vi "HeartRateControl_SMC+FF_New_Int.vi"() -> ()   [LabVIEW 2013]
uses:
  <vilib>/Instr/_visa.llb/VISA Configure Serial Port (Instr).vi
panel:
  out "Volt2":dbl
  out "Volt":dbl
  out "TM":dbl
  out "Torque [Nm]":dbl
  out "Cadence [rpm]":dbl
  out "Power [W]":dbl
  in  "file path":path
  out "Heart Rate [bpm]":u32
  out "Heart Rate [bpm]":dbl(knob) scale=0.0..220.0
  in  "VISA resource name":refnum<visa-resource-name>="COM1"
  out "Power [W]":dbl(slide) scale=0.0..250.0
  out "Cadence [rpm]":dbl(knob) scale=0.0..120.0
  out "Count":dbl
  out "Torque [Nm]":dbl(knob) scale=-250.0..250.0
  out "Torque [V]":dbl
  out "Sine":bool
  out "Cosine":bool
  in  "stop (F)":bool caption="Stop"
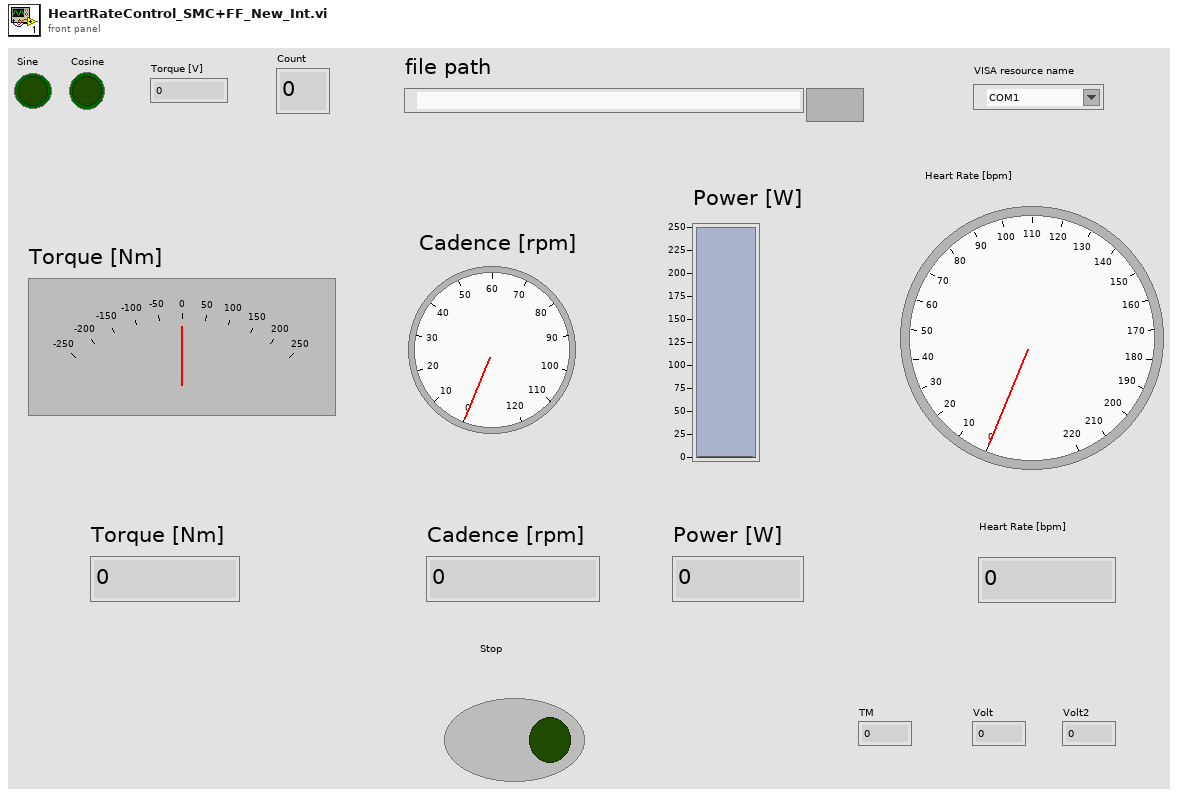
[diagram p1: front panel]
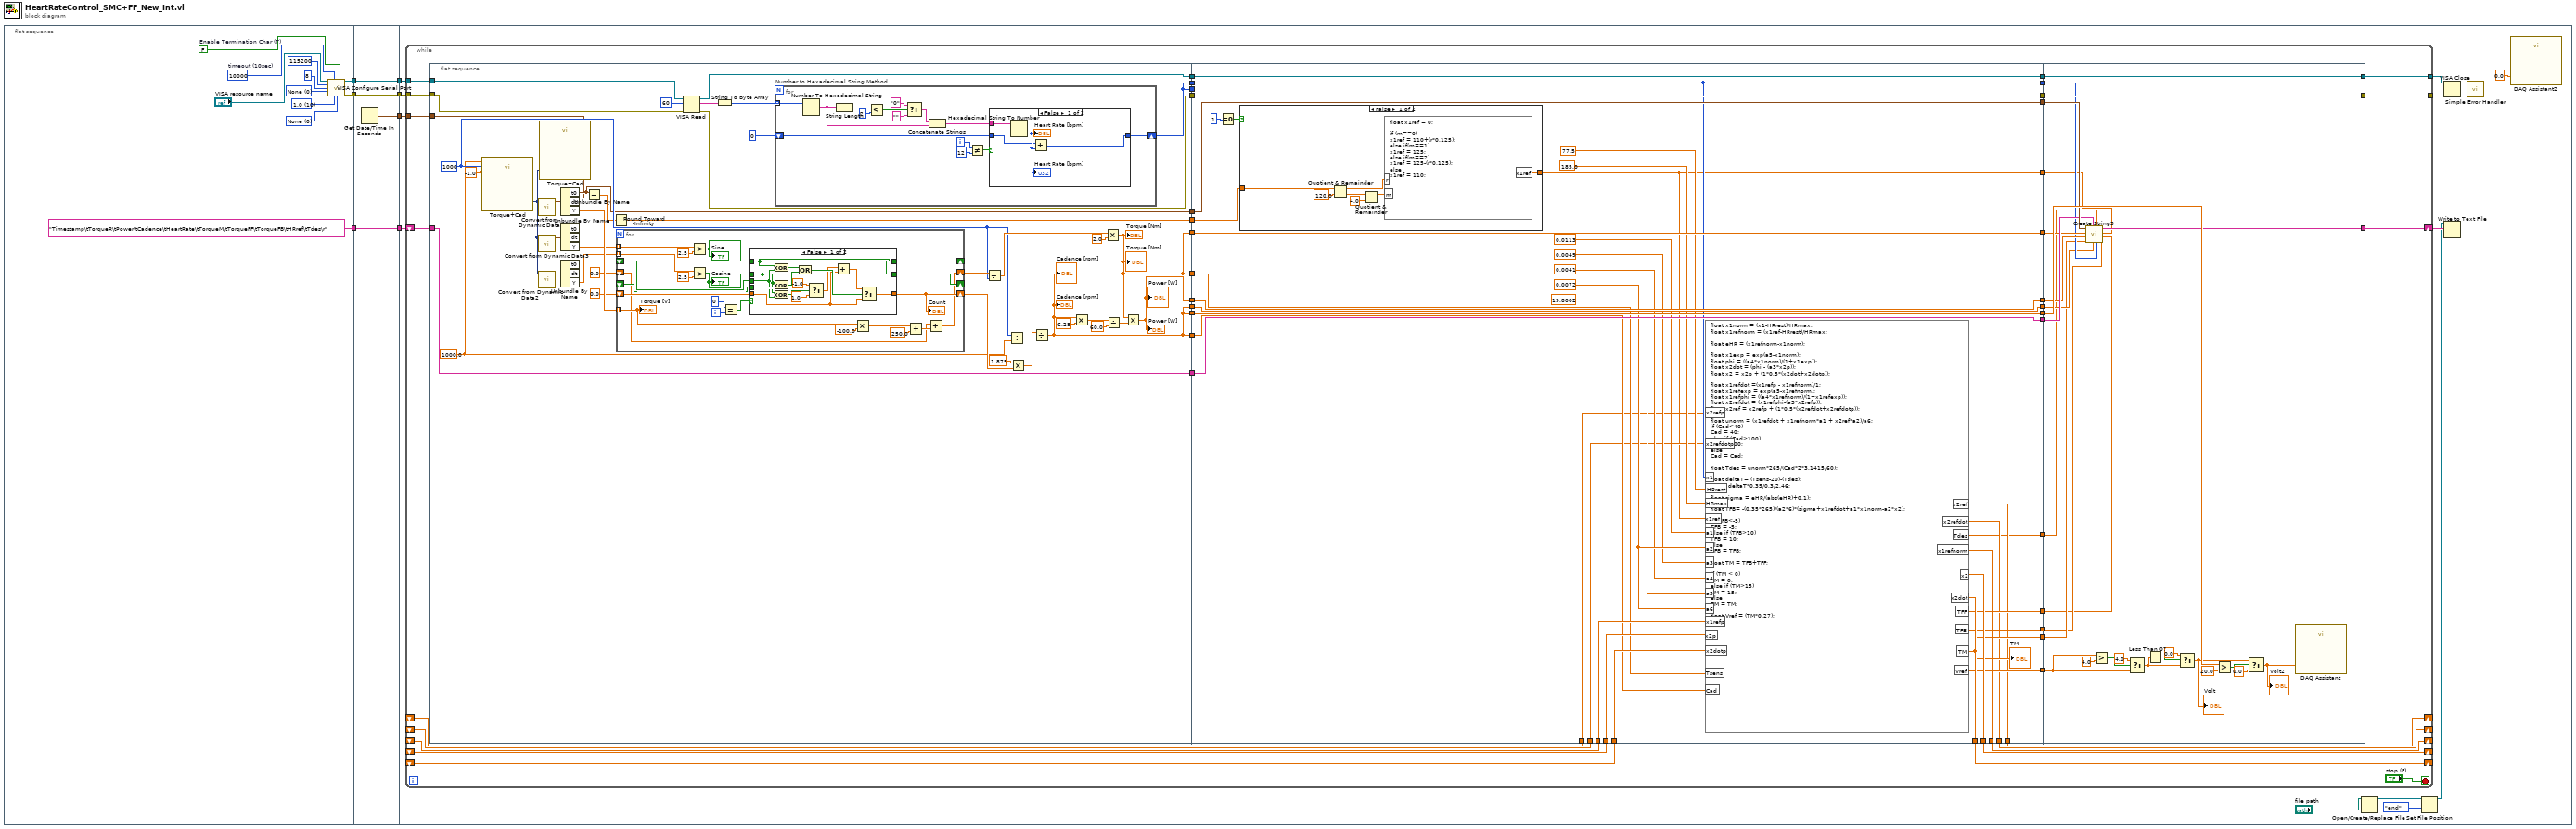
[diagram p0: block diagram]
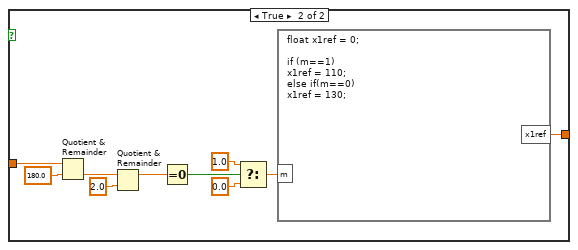
[diagram p4: hidden frame]
diagram:
  n1 = flat-sequence {
    tunnel: [w10] -> w6
    tunnel: [w9] -> w4
    tunnel: ["Timestamp\tTorqueR\tPower\tCadence\tHeartRate\tTorqueM\tTorqueFF\tTorqueFB\tHRref\tTdes\r" ("String out")] -> w2
    tunnel: [w22] -> w7
    tunnel: w6 -> [w22]
    tunnel: [w21] -> w5
    tunnel: w4 -> [w21]
    tunnel: [w20] -> w3
    tunnel: w2 -> [w20]
    tunnel: [w19] -> w1
    tunnel: w7 -> [w26]
    tunnel: w5 -> [w25]
    tunnel: w3 -> [w24]
    tunnel: w1 -> [w23]
    frame #0 {
      w16 = u16 0 items=["None"=0, "XON/XOFF"=1, "RTS/CTS"=2, "DTR/DSR"=4] ("flow control")
      w15 = u16 10 items=["1.0"=10, "1.5"=15, "2.0"=20] ("stop bits")
      w12 = u16 0 items=["None", "Odd", "Even", "Mark", "Space"] ("parity")
      w14 = FALSE  # Enable Termination Char (T)
      w13 = u32 10000  # timeout (10sec)
      n2 = call-poly "VISA Configure Serial Port"("VISA resource name"="VISA resource name", "timeout (10sec)"=w13, "Enable Termination\nChar (T)"=w14, "baud rate (9600)"=u32 115200, "data bits (8)"=u16 8, "parity (0:none)"=w12, "stop bits (10: 1 bit)"=w15, "flow control (0:none)"=w16) -> ("VISA resource name out"=w10:refnum<visa-resource-name>, "error out"=w9:errorcluster)  [unwired: 6 in]
    }
    frame #1 {
      n3 = Get Date/Time In Seconds() -> (seconds since 1Jan1904=w19:timestamp)
    }
    frame #2 {
      n4 = while {
        tunnel: w26 -> [w79]
        tunnel: w25 -> [w78]
        tunnel: [w77] -> w33
        tunnel: [w76] -> w32
        shift-right: [w75] -> w31
        shift-left: w24 -> [w74]
        shift-right: [w51] -> _
        shift-left: _ -> [w70]
        shift-right: [w50] -> _
        shift-left: _ -> [w69]
        shift-right: [w49] -> _
        shift-left: _ -> [w64]
        shift-right: [w42] -> _
        shift-left: _ -> [w41]
        shift-right: [w40] -> _
        shift-left: _ -> [w39]
        tunnel: w23 -> [w37]
        stop <- "stop (F)" stop-if-true
        n5 = flat-sequence {
          tunnel: w79 -> [w99]
          tunnel: w78 -> [w98]
          tunnel: w74 -> [w92]
          tunnel: [w97] -> w73
          tunnel: [w96] -> w72
          tunnel: [w90] -> w71
          tunnel: [w85] -> w65
          tunnel: [w84] -> w62
          tunnel: [w92] -> w60
          tunnel: [w86] -> w58
          tunnel: [w91] -> w56
          tunnel: [w90] -> w54
          tunnel: [w85] -> w52
          tunnel: [w86] -> w44
          tunnel: [w85] -> w43
          tunnel: w37 -> [w83]
          tunnel: [w81] -> w36
          tunnel: w73 -> [w215]
          tunnel: w72 -> [w214]
          tunnel: w71 -> [_]
          tunnel: w70 -> [w198]
          tunnel: w69 -> [w196]
          tunnel: [w215] -> w68
          tunnel: [w214] -> w67
          tunnel: [w213] -> w66
          tunnel: w65 -> [w213]
          tunnel: w64 -> [w194]
          tunnel: [w212] -> w63
          tunnel: w62 -> [w212]
          tunnel: [w211] -> w61
          tunnel: w60 -> [w211]
          tunnel: [w208] -> w59
          tunnel: w58 -> [w208]
          tunnel: [w210] -> w57
          tunnel: w56 -> [w210]
          tunnel: [w207] -> w55
          tunnel: w54 -> [w207]
          tunnel: [w209] -> w53
          tunnel: w52 -> [w209]
          tunnel: [w199] -> w51
          tunnel: [w197] -> w50
          tunnel: [w195] -> w49
          tunnel: [w193] -> w48
          tunnel: [w192] -> w47
          tunnel: [w191] -> w46
          tunnel: [w190] -> w45
          tunnel: w44 -> [w189]
          tunnel: w43 -> [w188]
          tunnel: [w187] -> w42
          tunnel: w41 -> [w186]
          tunnel: [w185] -> w40
          tunnel: w39 -> [w184]
          tunnel: [w183] -> w38
          tunnel: w36 -> [w182]
          tunnel: [w181] -> w35
          tunnel: [w245] -> w75
          tunnel: [w258] -> w76
          tunnel: [w259] -> w77
          tunnel: w68 -> [w259]
          tunnel: w67 -> [w258]
          tunnel: w66 -> [w248]
          tunnel: w63 -> [w244]
          tunnel: w61 -> [w243]
          tunnel: w59 -> [w242]
          tunnel: w57 -> [w241]
          tunnel: w55 -> [w240]
          tunnel: w53 -> [w239]
          tunnel: w48 -> [w238]
          tunnel: w47 -> [w235]
          tunnel: w46 -> [w237]
          tunnel: w45 -> [w236]
          tunnel: w38 -> [w234]
          tunnel: w35 -> [w233]
          frame #0 {
            w88 = 1000.0 ("rate")
            w89 = 1000 ("number of samples")
            n6 = call "Torque+Cad"("rate"=w88, "number of samples"=w89, "timeout (s)"=-1.0) -> ("data"=w117:dynamicdata)  [unwired: 14 in, 2 out]
            n7 = call "Convert from Dynamic Data"("Dynamic Data Type"=w117) -> ("Waveform"=w119:waveform(dbl))  [unwired: 3 in]
            n8 = call "Convert from Dynamic Data3"("Dynamic Data Type"=w117) -> ("Waveform"=w116:waveform(dbl))  [unwired: 3 in]
            n9 = call "Convert from Dynamic Data2"("Dynamic Data Type"=w117) -> ("Waveform"=w118:waveform(dbl))  [unwired: 3 in]
            n10 = call "Torque+Cad"("Signals"=w117) -> ()  [unwired: 16 in, 3 out]
            n11 = Unbundle By Name(w119) -> ("t0"=w84:timestamp, "Y"=w115:dbl[])  [unwired: 1 out]
            n12 = Unbundle By Name(w116) -> ("Y"=w113:dbl[])  [unwired: 2 out]
            n13 = Unbundle By Name(w118) -> ("Y"=w114:dbl[])  [unwired: 2 out]
            n14 = Subtract(x=w84, y=w83) -> (x-y=w82:dbl)
            n15 = Round Toward -Infinity(1:w82) -> (0:w81:dbl)
            n16 = for {
              tunnel: w115 -> [w159] mode=indexing
              tunnel: w114 -> [w141] mode=indexing
              tunnel: w113 -> [w140] mode=indexing
              shift-right: [w152] -> _
              shift-left: _ -> [w148]
              shift-right: [w150] -> _
              shift-left: _ -> [w147]
              shift-right: [w146] -> w109
              shift-left: 0.0 -> [w145]
              shift-right: [w143] -> w108
              shift-left: 0.0 -> [w142]
              i -> [w155]
              n17 = Greater?(x=w140, y=2.5) -> (0:w151:bool)
              "Sine" <- w151
              n18 = Greater?(x=w141, y=2.5) -> (0:w149:bool)
              "Cosine" <- w149
              n19 = Equal?(x=0, y=w155) -> (x = y?=w153:bool)
              n20 = case shown="False" w153 {
                tunnel: [w164 w178] -> w152
                tunnel: w151 -> [w164 w178]
                tunnel: [w163 w177] -> w150
                tunnel: w149 -> [w163 w177]
                tunnel: w148 -> [w172 _]
                tunnel: w147 -> [w175 _]
                tunnel: [w165 w176] -> w146
                tunnel: w145 -> [w162 w176]
                frame False {
                  n21 = Exclusive Or(1:w172, 2:w164) -> (0:w174:bool)
                  n22 = Exclusive Or(1:w175, 2:w163) -> (0:w173:bool)
                  n23 = Exclusive Or(1:w172, 2:w163) -> (0:w171:bool)
                  n24 = Or(x=w174, y=w173) -> (x .or. y?=w170:bool)
                  n25 = Select(t=-1.0, s=w171, f=1.0) -> (s? t:f=w167:dbl)
                  n26 = Add(x=w167, y=w162) -> (x+y=w166:dbl)
                  n27 = Select(t=w166, s=w170, f=w162) -> (s? t:f=w165:dbl)
                }
                frame True {
                }
              }
              "Count" <- w146
              n28 = Multiply(x=w159, y=-100.0) -> (x*y=w157:dbl)
              n29 = Add(x=w157, y=250.0) -> (x+y=w144:dbl)
              n30 = Add(x=w142, y=w144) -> (x+y=w143:dbl)
              "Torque [V]" <- w159
            }
            n31 = VISA Read(VISA resource name=w99, byte count=u32 60 ("bytes to read"), error in (no error)=w98) -> (VISA resource name out=w97:refnum<visa-resource-name>, read buffer=w101:string, error out=w96:errorcluster)  [unwired: 1 out]
            n32 = String To Byte Array(string=w101) -> (unsigned byte array=w100:u8[])
            n33 = for "Number to Hexadecimal String Method" {
              tunnel: w100 -> [w130] mode=indexing
              shift-right: [w122] -> w90
              shift-left: u32 0 -> [w121]
              i -> [w126]
              n34 = Number To Hexadecimal String(2:w130) -> (0:w127:string)  [unwired: 1 in]
              n35 = String Length(string=w127) -> (length=w134:i32)
              n36 = Less?(x=w134, y=2) -> (x < y?=w132:bool)
              n37 = Select(t="0", s=w132, f="") -> (s? t:f=w128:string)
              n38 = Concatenate Strings(w128, w127) -> (w123:string)
              n39 = Not Equal?(x=w126, y=12) -> (x != y?=w124:bool)
              n40 = case shown="False" w124 {
                tunnel: w123 -> [w138 _]
                tunnel: [w136 w139] -> w122
                tunnel: w121 -> [w135 w139]
                frame False {
                  n41 = Hexadecimal String To Number(string=w138) -> (number=w137:u32)  [unwired: 2 in, 1 out]
                  "Heart Rate [bpm]" <- w137
                  "Heart Rate [bpm]" <- w137
                  n42 = Add(x=w135, y=w137) -> (x+y=w136:u32)
                }
                frame True {
                }
              }
            }
            n43 = Divide(x=w108, y=w89) -> (x/y=w94:dbl)
            n44 = Divide(x=w89, y=w88) -> (x/y=w87:dbl)
            n45 = Multiply(x=1.875, y=w109) -> (x*y=w112:dbl)
            n46 = Divide(x=w112, y=w87) -> (x/y=w85:dbl)
            "Cadence [rpm]" <- w85
            "Cadence [rpm]" <- w85
            n47 = Multiply(x=w85, y=6.28) -> (x*y=w106:dbl)
            n48 = Multiply(x=w94, y=2.0) -> (x*y=w86:dbl)
            "Torque [Nm]" <- w86
            "Torque [Nm]" <- w86
            n49 = Divide(x=w106, y=60.0) -> (x/y=w104:dbl)
            n50 = Multiply(x=w86, y=w104) -> (x*y=w91:dbl)
            "Power [W]" <- w91
            "Power [W]" <- w91
          }
          frame #1 {
            w203 = 0.0072 ("input variable")
            n51 = Equal To 0?(x=1) -> (x = 0?=w179:bool)
            n52 = case shown="False" w179 {
              tunnel: [w222 w232] -> w181
              tunnel: w182 -> [w219 w225]
              frame False {
                n53 = Quotient & Remainder(x=w219, y=120.0) -> (x-y*floor(x/y)=w216:dbl, floor(x/y)=w218:dbl)
                n54 = Quotient & Remainder(x=w218, y=4.0) -> (x-y*floor(x/y)=w217:dbl)  [unwired: 1 out]
                n55 = formula code="float x1ref = 0;\n\nif (m==0)\nx1ref = 110+(r*0.125);\nelse if(m==1)\nx1ref = 125;\nelse if(m==2)\nx1ref = 125-(r*0.125);\nelse\nx1ref = 110;"("m"=w217, "r"=w216) -> ("x1ref"=w222:dbl)
              }
              frame True {
                n56 = Quotient & Remainder(x=w225, y=180.0) -> (floor(x/y)=w224:dbl)  [unwired: 1 out]
                n57 = Quotient & Remainder(x=w224, y=2.0) -> (x-y*floor(x/y)=w229:dbl)  [unwired: 1 out]
                n58 = Equal To 0?(x=w229) -> (x = 0?=w228:bool)
                n59 = Select(t=1.0, s=w228, f=0.0) -> (s? t:f=w223:dbl)
                n60 = formula code="float x1ref = 0;\n\nif (m==1)\nx1ref = 110;\nelse if(m==0)\nx1ref = 130;"("m"=w223) -> ("x1ref"=w232:dbl)
              }
            }
            n61 = formula code="float x1norm = (x1-HRrest)/HRmax;\nfloat x1refnorm = (x1ref-HRrest)/HRmax;\n\nfloat eHR = (x1refnorm-x1norm);\n\nfloat x1exp = exp(a5-x1norm);\nfloat phi = ((a4*x1norm)/(1+x1exp));\nfloat x2dot = (phi - (a3*x2p));\nfloat x2 = x2p + (1*0.5*(x2dot+x2dotp));\n\nfloat x1refdot =(x1refp - x1refnorm)/1;\nfloat x1refexp = exp(a5-x1refnorm);\nfloat x1refphi = ((a4*x1refnorm)/(1+x1refexp));\nfloat x2refdot = (x1refphi-(a3*x2refp));\nfloat x2ref = x2refp + (1*0.5*(x2refdot+x2refdotp));\n\nfloat unorm = (x1refdot + x1refnorm*a1 + x2ref*a2)/a6;\nif (Cad<40)\nCad = 40;\nelse if (Cad>100)\nCad = 100;\nelse\nCad = Cad;\n\nfloat Tdes = unorm*265/(Cad*2*3.1415/60);\n\nfloat deltaT= (Tsens-20)-(Tdes);\nTFF = deltaT*0.35/0.3/2.46;\n\nfloat sigma = eHR/(abs(eHR)+0.1);\n\nfloat TFB= -(0.35*265)/(a2*6)*(sigma+x1refdot+a1*x1norm-a2*x2);\n\nif (TFB<-5)\nTFB = -5;\nelse if (TFB>10)\nTFB = 10;\nelse\nTFB = TFB;\n\nfloat TM = TFB+TFF;\n\nif (TM < 0)\nTM = 0;\nelse if (TM>15)\nTM = 15;\nelse\nTM = TM;\n\nfloat Vref = (TM*0.27);"("HRrest"=77.5 ("y"), "x1"=w207, "HRmax"=185.0 ("y"), "x1ref"=w181, "a1"=0.0113 ("input variable"), "a2"=w203, "a3"=0.0049 ("input variable"), "a4"=0.0041 ("input variable"), "a5"=19.8002 ("x"), "a6"=w203, "x1refp"=w198, "x2p"=w196, "x2dotp"=w194, "Tsens"=w189, "Cad"=w188, "x2refp"=w186, "x2refdotp"=w184) -> ("x1refnorm"=w199:dbl, "x2"=w197:dbl, "x2dot"=w195:dbl, "TFF"=w190:dbl, "TFB"=w191:dbl, "TM"=w193:dbl, "Vref"=w192:dbl, "x2ref"=w187:dbl, "x2refdot"=w185:dbl, "Tdes"=w183:dbl)
            "TM" <- w193
          }
          frame #2 {
            n62 = call "Create String3.vi"("Torque FB"=w237, "Torque FF"=w236, "HRref"=w233, "Heart Rate"=w240, "Tdes"=w234, "Cadence"=w239, "String in"=w243, "Torque Motor"=w238, "Power"=w241, "Torque Rider"=w242, "t0"=w244) -> ("String out"=w245:string)
            n63 = Greater?(x=w235, y=4.0) -> (0:w256:bool)
            n64 = Select(t=4.0, s=w256, f=w235) -> (s? t:f=w252:dbl)
            n65 = Less Than 0?(x=w252) -> (x < 0?=w254:bool)
            n66 = Select(t=0.0, s=w254, f=w252) -> (s? t:f=w246:dbl)
            "Volt" <- w246
            n67 = Greater?(x=w248, y=20.0) -> (0:w250:bool)
            n68 = Select(t=w246, s=w250, f=0.0) -> (s? t:f=w247:dbl)
            "Volt2" <- w247
            n69 = call "DAQ Assistant"("data"=w247) -> ()  [unwired: 17 in, 2 out]
          }
        }
      }
      n70 = Open/Create/Replace File(file path (use dialog)="file path") -> (refnum out=w29:refnum<file>)  [unwired: 5 in, 2 out]
      n71 = Set File Position(refnum=w29, from (0:start)=enum16{"start", "end", "current"}."end") -> (refnum out=w28:refnum<file>)  [unwired: 2 in, 1 out]
      n72 = VISA Close(VISA resource name=w33, error in (no error)=w32) -> (error out=w34:errorcluster)
      n73 = Write to Text File(file (use dialog)=w28, text=w31) -> ()  [unwired: 2 in, 3 out]
      n74 = call <vilib>:"Simple Error Handler.vi"("error in (no error)"=w34) -> ()  [unwired: 4 in, 5 out]
    }
    frame #3 {
      n75 = call "DAQ Assistant2"("data"=0.0) -> ()  [unwired: 17 in, 2 out]
    }
  }
